vi "ReadIVIsampleFGEN.vi"(0 "logical name (\"SampleFGen\")":string="SampleFGen") -> (1 "instrument handle":refnum<k15>, 2 "channel name (\"CHANNEL1\")":string, 3 "error in (no error)":errorcluster)   [LabVIEW 2013]
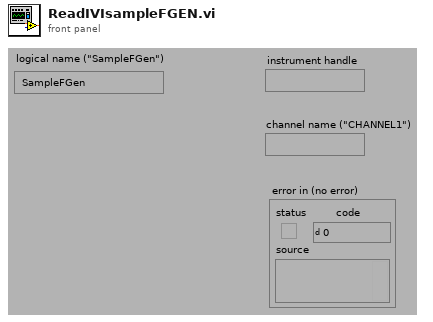
[diagram p1: front panel]
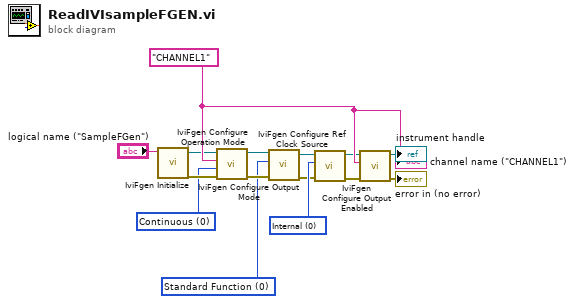
[diagram p0: block diagram]
diagram:
  w14 = "CHANNEL1" ("channel name (\"CHANNEL1\")")
  w2 = 0 items=["Continuous", "Burst"] ("operation mode (Continuous)")
  w4 = 0 items=["Standard Function", "Arbitrary Waveform", "Arbitrary Sequence"] ("output mode (Standard Function)")
  w9 = 0 items=["Internal"=0, "External"=1, "RTSI Clock"=101] ("reference clock source (Internal)")
  n1 = call <vilib>:"IviFgen Initialize.vi"("logical name (\"SampleFGen\")"="logical name (\"SampleFGen\")") -> ("error out"=w3:errorcluster, "instrument handle out"=w1:refnum<k15>)  [unwired: 3 in, 6 out]
  n2 = call <vilib>:"IviFgen Configure Operation Mode.vi"("error in (no error)"=w3, "operation mode (Continuous)"=w2, "channel name (\"CHANNEL1\")"=w14, "instrument handle"=w1) -> ("error out"=w5:errorcluster, "instrument handle out"=w6:refnum<k15>)  [unwired: 6 out]
  n3 = call <vilib>:"IviFgen Configure Output Mode.vi"("error in (no error)"=w5, "output mode (Standard Function)"=w4, "instrument handle"=w6) -> ("error out"=w7:errorcluster, "instrument handle out"=w8:refnum<k15>)  [unwired: 7 out]
  n4 = call <vilib>:"IviFgen Configure Ref Clock Source.vi"("error in (no error)"=w7, "reference clock source (Internal)"=w9, "instrument handle"=w8) -> ("error out"=w11:errorcluster, "instrument handle out"=w12:refnum<k15>)  [unwired: 7 out]
  n5 = call <vilib>:"IviFgen Configure Output Enabled.vi"("error in (no error)"=w11, "channel name (\"CHANNEL1\")"=w14, "instrument handle"=w12) -> ("error out"=→"error in (no error)":errorcluster, "instrument handle out"=→"instrument handle":refnum<k15>)  [unwired: 1 in, 6 out]
  "channel name (\"CHANNEL1\")" <- w14
